vi "Stop Core.vi"(10 "final error code":i32, 11 "WebSocket Service Actor in":refnum<class "WebSocket Service.lvclass">) -> (3 "WebSocket Service Actor out":refnum<class "WebSocket Service.lvclass">)   [LabVIEW 2021, in "WebSocket Actors.lvlib" / "WebSocket Service.lvclass"]
doc: "(<B>Filename</B>: Actor Framework.lvlib:Actor.lvclass:Stop Core.vi)\n\nDefines what the actor does before it stops. Use the <B>final error code</B> input to determine whether the actor shut down in response to an error.\n\nBy default, this method does nothing. A descendant class may override it to define behavior, such as shutting down any processes the actor initiated in its override of the Actor Core method."
uses:
  WebSocket Service.lvclass
  WebSocket Service.lvclass/WebSocket Service.ctl
  <vilib>/ActorFramework/Message Enqueuer/Message Enqueuer.lvclass
  <vilib>/ActorFramework/Message Enqueuer/Message Enqueuer.lvclass/Message Enqueuer.ctl
  <vilib>/ActorFramework/Message Enqueuer/Enqueue.vi
  <vilib>/ActorFramework/Stop Msg/Stop Msg.lvclass
  C:/Program Files/National Instruments/LabVIEW 2021/vi.lib/ActorFramework/Message/Message.lvclass
  <vilib>/Utility/LVClass/Get LV Class Name.vi
  <resource>/AFDebug/Generate Trace for Message.vi
  <vilib>/ActorFramework/Message Priority Queue/Priority Enqueue.vi
  <vilib>/ActorFramework/Actor/Actor.lvclass
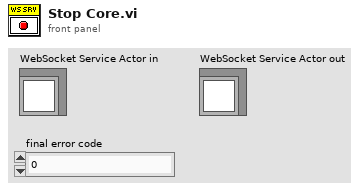
[diagram p1: front panel]
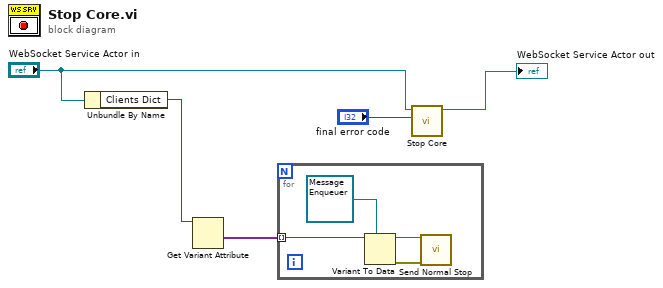
[diagram p0: block diagram]
diagram:
  n1 = Unbundle By Name("WebSocket Service Actor in") -> ("Clients Dict"=w2:variant)
  n2 = Get Variant Attribute(Variant=w2) -> (values=w1:variant[])  [unwired: 3 in, 3 out]
  n3 = for {
    tunnel: w1 -> [w8] mode=indexing
    n4 = Variant To Data(type=refnum<class "Message Enqueuer.lvclass"> refnum ("Message Enqueuer in"), Variant=w8) -> (data=w7:refnum<class "Message Enqueuer.lvclass">, error out=w6:errorcluster)  [unwired: 1 in]
    n5 = call <vilib>:"Send Normal Stop.vi"("error in (no error)"=w6, "Message Enqueuer"=w7) -> ()  [unwired: 9 in, 1 out]
  }
  n6 = call-parent "Stop Core.vi"("final error code"="final error code", "Actor in"="WebSocket Service Actor in") -> ("Actor out"=→"WebSocket Service Actor out":refnum<class "WebSocket Service.lvclass">)  [unwired: 9 in]
